vi "oa_SCL Calc Corrdinate.vi"(9 "scale info":T1, 11 "cursor list":T2 {"Location"."Y" format="%.2f"; "Location"."X" format="%.2f"}) -> (1 "position":cluster{"x":i16, "y":i16}, 3 "Name":string)   [LabVIEW 2017]
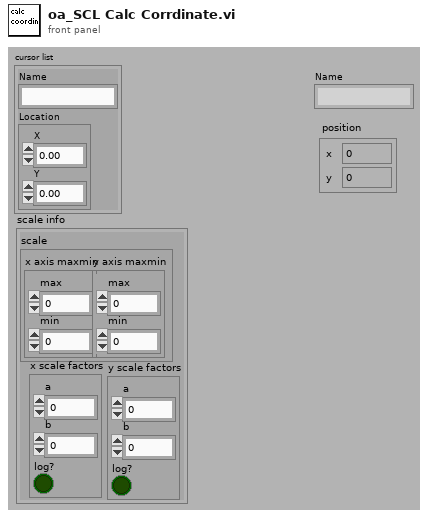
[diagram p1: front panel]
types:
  T1 = cluster{"scale":cluster{"x axis maxmin":cluster{"max":dbl, "min":dbl}, "y axis maxmin":cluster{"max":dbl, "min":dbl}}, "x scale factors":cluster{"a":dbl, "b":dbl, "log?":bool}, "y scale factors":cluster{"a":dbl, "b":dbl, "log?":bool}}
  T2 = cluster{"Name":string, "Location":cluster{"X":dbl, "Y":dbl}}
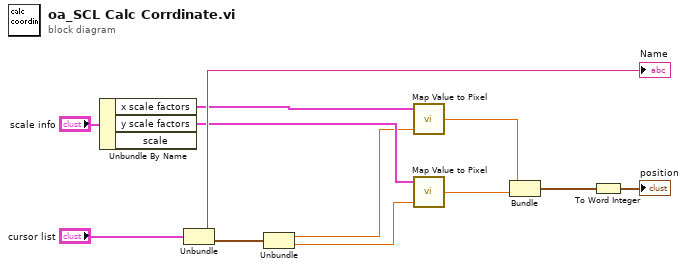
[diagram p0: block diagram]
diagram:
  n1 = Unbundle By Name("scale info") -> ("x scale factors"=w8:cluster{"a":dbl, "b":dbl, "log?":bool}, "y scale factors"=w7:cluster{"a":dbl, "b":dbl, "log?":bool})  [unwired: 1 out]
  n2 = Unbundle("cursor list") -> ("Name"=→"Name":string, "Location"=w10:cluster{"X":dbl, "Y":dbl})
  n3 = Unbundle(w10) -> ("X"=w2:dbl, "Y"=w1:dbl)
  n4 = call <vilib>:"Map Value to Pixel.vi"("x"=w2, "scale factors"=w8) -> ("pixel"=w6:dbl)  [unwired: 1 in]
  n5 = call <vilib>:"Map Value to Pixel.vi"("x"=w1, "scale factors"=w7) -> ("pixel"=w5:dbl)  [unwired: 1 in]
  n6 = Bundle("pixel"=w6, "pixel"=w5) -> (w3:cluster{"pixel":dbl, "pixel":dbl})  [unwired: 1 in]
  n7 = To Word Integer(number=w3) -> (16bit integer=→"position":cluster{"pixel":i16, "pixel":i16})
